vi "elevated buttons.vi"(9 "control-level":string, 11 "Material-Scheme in":refnum<class "Material-Scheme.lvclass">) -> (1 "font color":u32(colorbox), 2 "colors array":cluster{"bg":u32, "fg":u32}[](array[cluster]))   [LabVIEW 2021, in "TSC Material Theme.lvlib" / "Material-Scheme.lvclass"]
doc: "application of the floating action button transparent buttons (text buttons) rules\n\nhttps://m3.material.io/components/buttons/specs#9c12a1a1-9a74-499c-8139-5cff551afe4f\n\n<b>Code Developed By:</b>\nTechnology Service Corporation\nwww.tsc.com/atcs\n\nDeveloper:\nDaniel Coons"
uses:
  Material-Scheme.lvclass
  Material-Scheme.lvclass/Material-Scheme.ctl
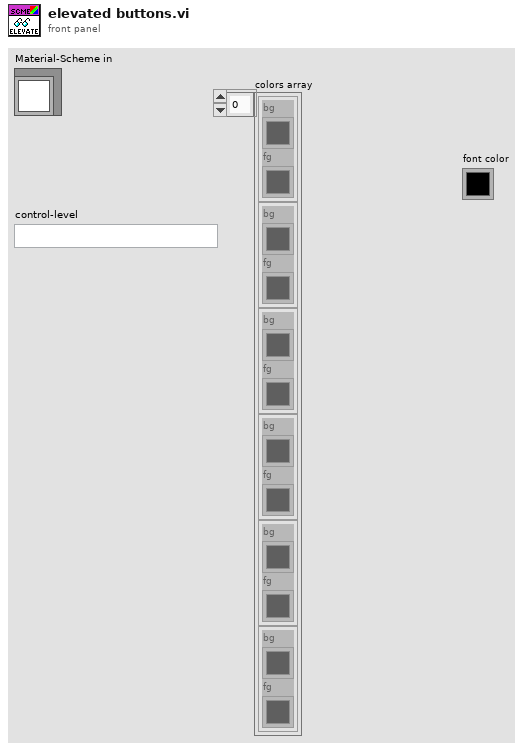
[diagram p1: front panel]
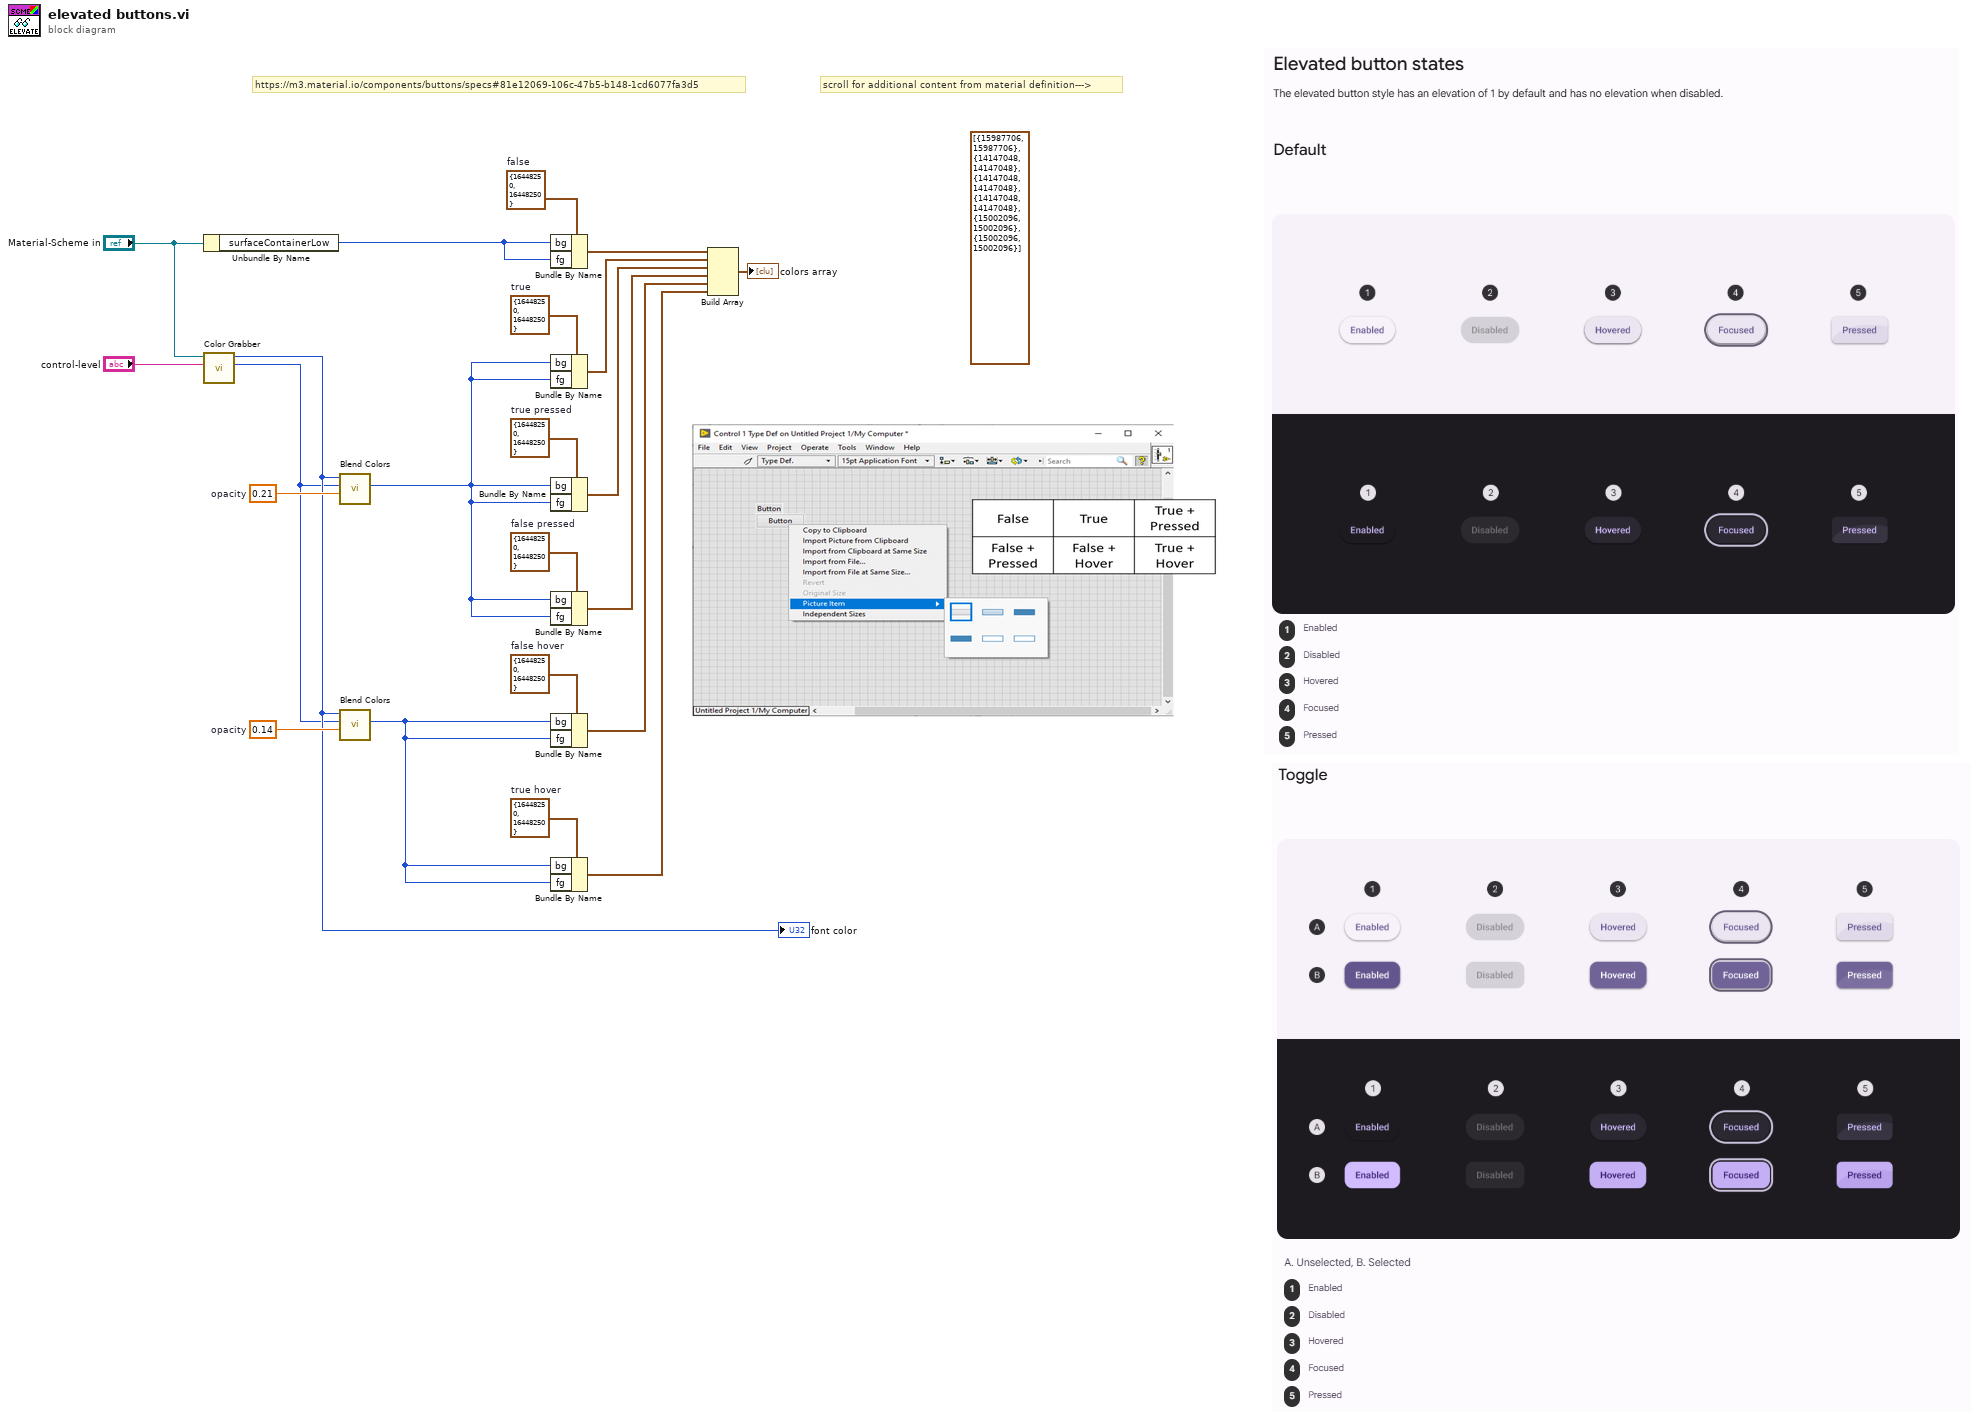
[diagram p0: block diagram]
diagram:
  (unwired) cluster{"bg":u32, "fg":u32}[] [{"bg"=15987706, "fg"=15987706}, {"bg"=14147048, "fg"=14147048}, {"bg"=14147048, "fg"=14147048}, {"bg"=14147048, "fg"=14147048}, {"bg"=15002096, "fg"=15002096}, {"bg"=15002096, "fg"=15002096}] ("colors array 2")
  w6 = 0.14  # opacity
  w7 = 0.21  # opacity
  w17 = cluster{"bg":u32, "fg":u32} {"bg"=16448250, "fg"=16448250}  # true hover
  w18 = cluster{"bg":u32, "fg":u32} {"bg"=16448250, "fg"=16448250}  # false hover
  w19 = cluster{"bg":u32, "fg":u32} {"bg"=16448250, "fg"=16448250}  # false pressed
  w20 = cluster{"bg":u32, "fg":u32} {"bg"=16448250, "fg"=16448250}  # true pressed
  w21 = cluster{"bg":u32, "fg":u32} {"bg"=16448250, "fg"=16448250}  # true
  w22 = cluster{"bg":u32, "fg":u32} {"bg"=16448250, "fg"=16448250}  # false
  # "https://m3.material.io/components/buttons/specs#81e12069-106c-47b5-b148-1cd6077fa3d5"
  # "scroll for additional content from material definition--->"
  n1 = Unbundle By Name("Material-Scheme in") -> ("surfaceContainerLow"=w1:u32)
  n2 = call "Color Grabber.vi"("control-level"="control-level", "Material-Scheme in"="Material-Scheme in") -> ("onColor"=w2:u32, "color"=w3:u32)  [unwired: 3 in, 5 out]
  "font color" <- w3
  n3 = call "Blend Colors.vi"("blend ratio"=w7, "onColor"=w2, "Color"=w3) -> ("Modified Color"=w4:u32)  [unwired: 8 in]
  n4 = call "Blend Colors.vi"("blend ratio"=w6, "onColor"=w2, "Color"=w3) -> ("Modified Color"=w5:u32)  [unwired: 8 in]
  n5 = Bundle By Name(cluster=w22, "bg"=w1, "fg"=w1) -> (w16:cluster{"bg":u32, "fg":u32})
  n6 = Bundle By Name(cluster=w21, "bg"=w4, "fg"=w4) -> (w15:cluster{"bg":u32, "fg":u32})
  n7 = Bundle By Name(cluster=w20, "bg"=w4, "fg"=w4) -> (w14:cluster{"bg":u32, "fg":u32})
  n8 = Bundle By Name(cluster=w19, "bg"=w4, "fg"=w4) -> (w13:cluster{"bg":u32, "fg":u32})
  n9 = Bundle By Name(cluster=w18, "bg"=w5, "fg"=w5) -> (w12:cluster{"bg":u32, "fg":u32})
  n10 = Bundle By Name(cluster=w17, "bg"=w5, "fg"=w5) -> (w11:cluster{"bg":u32, "fg":u32})
  n11 = Build Array(w16, w15, w14, w13, w12, w11) -> (→"colors array":cluster{"bg":u32, "fg":u32}[])
